vi "Analog Output Sound.vi"(9 "rate":dbl=23000.0, 10 "Sound File":path, 11 "physical channels":tag) -> ()   [LabVIEW 2011]
uses:
  <vilib>/Utility/error.llb/DialogType.ctl
  <vilib>/DAQmx/write.llb/DAQmx Write (Analog 1D DBL 1Chan NSamp).vi
  <vilib>/DAQmx/create/channels.llb/DAQmx Create Channel (AO-Voltage-Basic).vi
  <vilib>/DAQmx/configure/timing.llb/DAQmx Timing (Sample Clock).vi
  <vilib>/DAQmx/miscellaneous.llb/DAQmx Fill In Error Info.vi
  C:/Program Files (x86)/National Instruments/LabVIEW 2011/resource/objmgr/daqmx.rc
panel:
  out "Sound Wave":waveform(dbl)(graph)
  in  "stop":bool
  # "Example can be found here:\nhttps://decibel.ni.com/content/docs/DOC-22121"
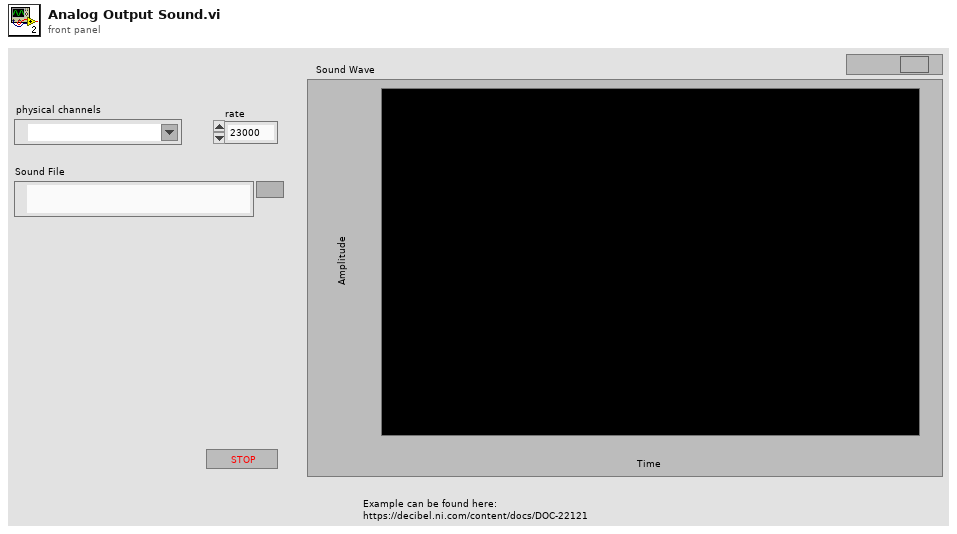
[diagram p1: front panel]
types:
  T1 = typedef "DialogType.ctl" = u16
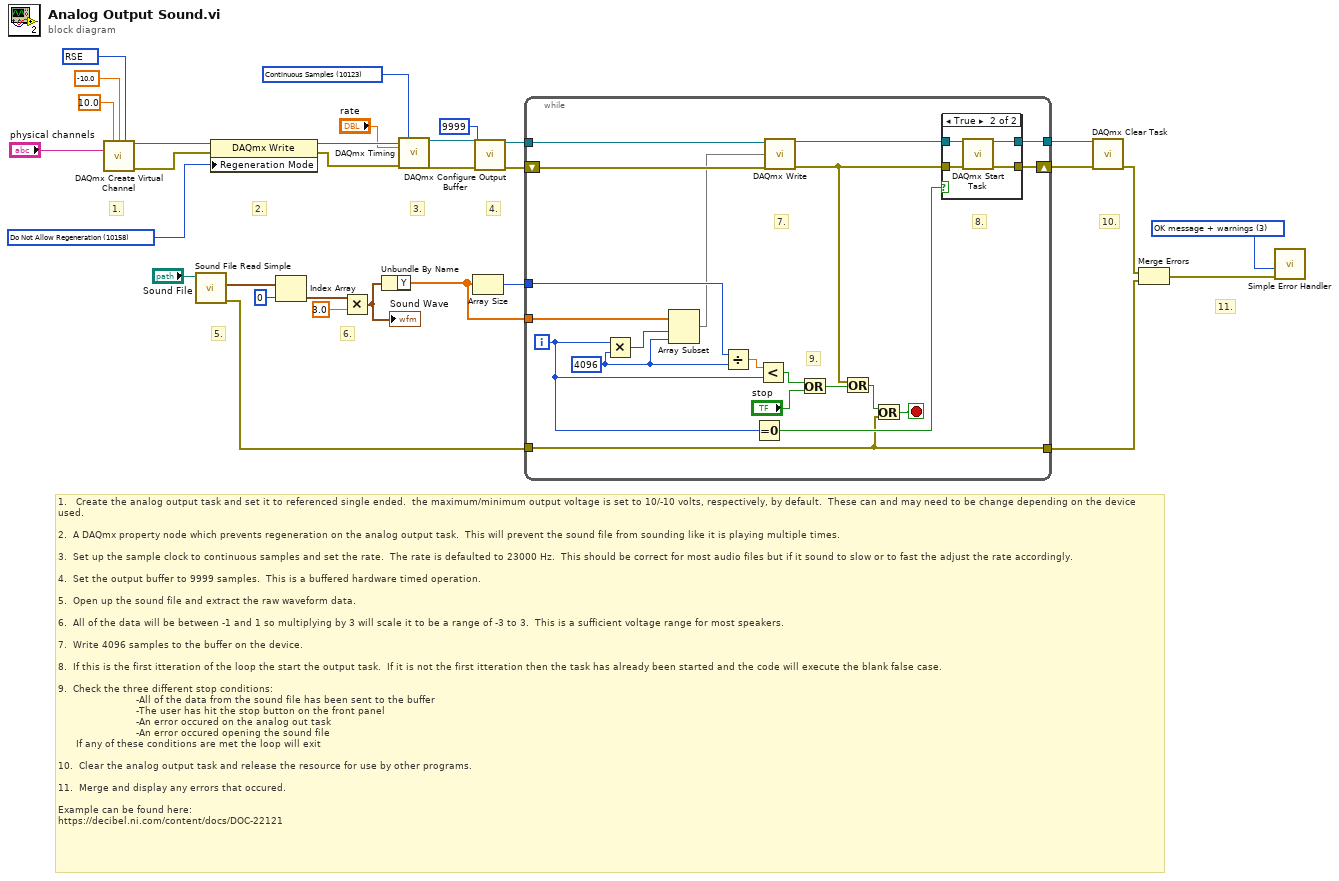
[diagram p0: block diagram]
diagram:
  w10 = T1 3 items=["no dialog", "OK message", "continue or stop message", "OK message + warnings", "continue/stop + warnings"] ("type of dialog (OK msg:1)")
  w15 = 10158 items=["Allow Regeneration"=10097, "Do Not Allow Regeneration"=10158] ("RegenMode")
  w21 = 10123 items=["Finite Samples"=10178, "Continuous Samples"=10123, "Hardware Timed Single Point"=12522] ("sample mode")
  w24 = 10083 items=["Default"=-1, "RSE"=10083, "Differential"=10106, "Pseudodifferential"=12529] ("output terminal configuration")
  # "1.   Create the analog output task and set it to referenced single ended.  the maximum/minimum output voltage is set to 10/-10 volts, respectively, by default.  These can and may need to be change depending on the device used.\n\n2.  A DAQmx property node which prevents regeneration on the analog output task.  This will prevent the sound file from sounding like it is playing multiple times.\n\n3.  Set up the sample clock to continuous samples and set the rate.  The rate is defaulted to 23000 Hz.  This should be correct for most audio files but if it sound to slow or to fast the adjust the rate accordingly.\n\n4.  Set the output buffer to 9999 samples.  This is a buffered hardware timed operation.\n\n5.  Open up the sound file and extract the raw waveform data.\n\n6.  All of the data will be between -1 and 1 so multiplying by 3 will scale it to be a range of -3 to 3.  This is a sufficient voltage range for most speakers. \n\n7.  Write 4096 samples to the buffer on the device.\n\n8.  If this is the first itteration of the loop the start the output task.  If it is not the first itteration then the task has already been started and the code will execute the blank false case.\n\n9.  Check the three different stop conditions:\n                          -All of the data from the sound file has been sent to the buffer\n                          -The user has hit the stop button on the front panel\n                          -An error occured on the analog out task\n                          -An error occured opening the sound file\n      If any of these conditions are met the loop will exit\n\n10.  Clear the analog output task and release the resource for use by other programs.\n\n11.  Merge and display any errors that occured.\n\nExample can be found here:\nhttps://decibel.ni.com/content/docs/DOC-22121"
  # "11."
  # "10."
  # "6."
  # "5."
  # "4."
  # "3."
  # "2."
  # "1."
  n1 = call-poly <vilib>:"DAQmx Create Virtual Channel.vi"("maximum value"=10.0, "minimum value"=-10.0, "output terminal configuration"=w24, "physical channels"="physical channels") -> ("task out"=w19:refnum<k21>, "error out"=w18:errorcluster)  [unwired: 10 in]
  n2 = call <vilib>:"Sound File Read Simple.vi"("path"="Sound File") -> ("error out"=w3:errorcluster, "data"=w7:waveform(dbl)[])  [unwired: 7 in, 2 out]
  n3 = property class="DAQmx Write"(reference=w19, error in=w18, "Regeneration Mode"=w15) -> (reference out=w17:refnum<k21>, error out=w16:errorcluster)
  n4 = Index Array(array=w7, index=0) -> (element=w29:waveform(dbl))
  n5 = Multiply(x=w29, y=3.0) -> (x*y=w27:waveform(dbl))
  "Sound Wave" <- w27
  n6 = Unbundle By Name(w27) -> ("Y"=w1:dbl[])
  n7 = call-poly <vilib>:"DAQmx Timing.vi"("task/channels in"=w17, "sample mode"=w21, "rate"="rate", "error in"=w16) -> ("task out"=w23:refnum<k21>, "error out"=w22:errorcluster)  [unwired: 10 in]
  n8 = Array Size(array=w1) -> (size(s)=w28:i32)
  n9 = call <vilib>:"DAQmx Configure Output Buffer.vi"("task/channels in"=w23, "buffer size (in samples per channel)"=u32 9999, "error in"=w22) -> ("task out"=w14:refnum<k21>, "error out"=w13:errorcluster)  [unwired: 11 out]
  n10 = while {
    tunnel: w28 -> [w48]
    tunnel: w1 -> [w51]
    tunnel: w14 -> [w44]
    tunnel: [w41] -> w12
    shift-right: [w40] -> w11
    shift-left: w13 -> [w43]
    tunnel: w3 -> [w32]
    tunnel: [w32] -> w2
    i -> [w38]
    stop <- w33 stop-if-true
    w49 = 4096
    # "9."
    # "8."
    # "7."
    n11 = Multiply(x=w38, y=w49) -> (x*y=w50:i32)
    n12 = Array Subset(array=w51, index=w50, length=w49) -> (w39:dbl[])
    n13 = Divide(x=w48, y=w49) -> (x/y=w47:dbl)
    n14 = Equal To 0?(x=w38) -> (x = 0?=w37:bool)
    n15 = Less?(x=w47, y=w38) -> (x < y?=w46:bool)
    n16 = call-poly <vilib>:"DAQmx Write.vi"("task/channels in"=w44, "data"=w39, "error in"=w43) -> ("task out"=w42:refnum<k21>, "error out"=w35:errorcluster)  [unwired: 10 in, 1 out]
    n17 = Or(x=w46, y="stop") -> (x .or. y?=w36:bool)
    n18 = Or(x=w35, y=w36) -> (x .or. y?=w34:bool)
    n19 = Or(x=w34, y=w32) -> (x .or. y?=w33:bool)
    n20 = case shown="True" w37 {
      tunnel: [w53 w57] -> w41
      tunnel: [w52 w56] -> w40
      tunnel: w42 -> [w53 w55]
      tunnel: w35 -> [w52 w54]
      frame False {
      }
      frame True {
        n21 = call <vilib>:"DAQmx Start Task.vi"("task/channels in"=w55, "error in"=w54) -> ("task out"=w57:refnum<k21>, "error out"=w56:errorcluster)  [unwired: 12 in]
      }
    }
  }
  n22 = call <vilib>:"DAQmx Clear Task.vi"("task in"=w12, "error in"=w11) -> ("error out"=w5:errorcluster)  [unwired: 13 in]
  n23 = Merge Errors(w5, w2) -> (w4:errorcluster)
  n24 = call <vilib>:"Simple Error Handler.vi"("type of dialog (OK msg:1)"=w10, "error in (no error)"=w4) -> ()  [unwired: 3 in, 5 out]
